vi "Post-Build Action.vi"(5 "Files Generated by Build":path[](array[path]), 6 "Top Level/Always Included VIs":path[](array[path]), 7 "Destination Path":path, 8 "error in (no error)":errorcluster, 9 "Target Name":string, 10 "Build Specification Name":string, 11 "Project Path":path) -> (0 "error out":errorcluster)   [LabVIEW 2016]
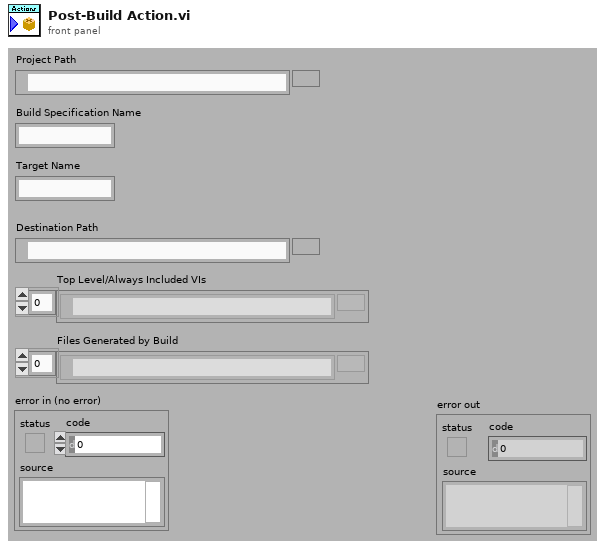
[diagram p1: front panel]
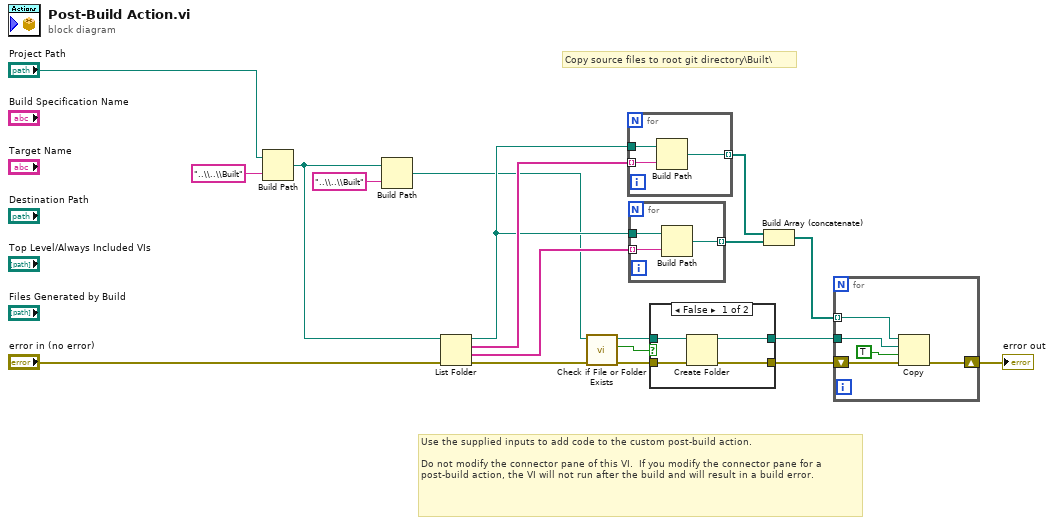
[diagram p0: block diagram]
diagram:
  # "Copy source files to root git directory\\Built\\"
  # "Use the supplied inputs to add code to the custom post-build action.\n\nDo not modify the connector pane of this VI.  If you modify the connector pane for a post-build action, the VI will not run after the build and will result in a build error."
  n1 = Build Path(base path="Project Path", name or relative path="..\\..\\Built") -> (appended path=w1:path)
  n2 = Build Path(base path=w1, name or relative path="..\\..\\Built") -> (appended path=w2:path)
  n3 = List Folder(path=w1, error in="error in (no error)") -> (path out=w12:path, filenames=w19:string[], folder names=w13:string[], error out=w10:errorcluster)  [unwired: 2 in]
  n4 = call <vilib>:"Check if File or Folder Exists.vi"("error in (no error)"=w10, "path"=w2) -> ("error out"=w14:errorcluster, "file or folder exists?"=w16:bool, "dup path"=w15:path)  [unwired: 7 in]
  n5 = for {
    tunnel: w19 -> [w21] mode=indexing
    tunnel: w12 -> [w22]
    tunnel: [w20] -> w18 mode=indexing
    n6 = Build Path(base path=w22, name or relative path=w21) -> (appended path=w20:path)
  }
  n7 = for {
    tunnel: w13 -> [w24] mode=indexing
    tunnel: w12 -> [w25]
    tunnel: [w23] -> w11 mode=indexing
    n8 = Build Path(base path=w25, name or relative path=w24) -> (appended path=w23:path)
  }
  n9 = case shown="False" w16 {
    tunnel: w15 -> [w29 w31]
    tunnel: w14 -> [w28 w30]
    tunnel: [w27 w31] -> w9
    tunnel: [w26 w30] -> w8
    frame False {
      n10 = Create Folder(path (use dialog)=w29, error in=w28) -> (created path=w27:path, error out=w26:errorcluster)  [unwired: 1 in, 1 out]
    }
    frame True {
    }
  }
  n11 = Build Array (concatenate)(w18, w11) -> (w17:path[])
  n12 = for {
    tunnel: w17 -> [w33] mode=indexing
    shift-right: [w34] -> w3
    shift-left: w8 -> [w35]
    tunnel: w9 -> [w32]
    n13 = Copy(8:w35, 9:TRUE ("overwrite (F)"), 10:w32, 11:w33) -> (0:w34:errorcluster)  [unwired: 1 in, 2 out]
  }
  "error out" <- w3
